vi "GT Ln XYG0.vi"(4 "fifo":i16, 5 "synAcc":dbl, 6 "synVel":dbl, 7 "y":i32, 8 "error in (no error)":errorcluster caption="错误输入（无错误）", 9 "x":i32, 10 "crd":i16, 11 "cardNum":i16) -> (0 "error out":errorcluster caption="错误输出", 3 "function return":i16)   [LabVIEW 2014, in "gts.lvlib"]
doc: "GT_API GT_LnXYG0(short cardNum,short crd,long x,long y,double synVel,double synAcc,short fifo=0);"
uses:
  gts.lvlib
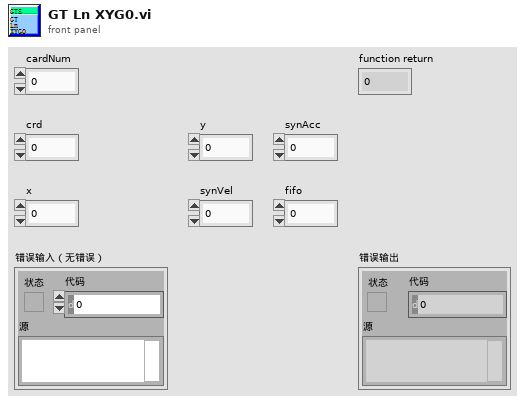
[diagram p1: front panel]
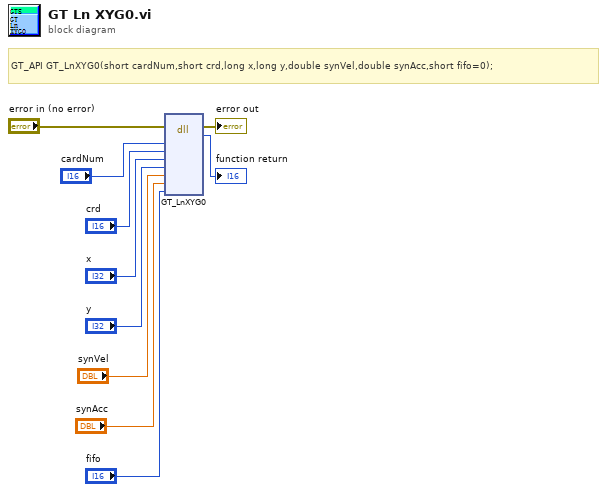
[diagram p0: block diagram]
diagram:
  # "GT_API GT_LnXYG0(short cardNum,short crd,long x,long y,double synVel,double synAcc,short fifo=0);"
  n1 = dll-call lib="PTH2habs D固高科技资料GTS控制卡GTS卡18年上半年资料dllVC32bit\nmulti_cardgts.*" fn="GT_LnXYG0"(error in="error in (no error)", "cardNum"="cardNum", "crd"="crd", "x"="x", "y"="y", "synVel"="synVel", "synAcc"="synAcc", "fifo"="fifo") -> (error out=→"error out":errorcluster, →"function return":i16)  [unwired: 9 in, 1 out]
